vi "PDLM_DecodeLHFeatures.vi"(8 "error in (no error)":errorcluster, 10 "features":u32) -> (0 "error out":errorcluster, 2 "Buffer":string, 3 "return type":i32)   [LabVIEW 2019]
uses:
  <userlib>/TaikoLaser/PDLM_DllPath_global.vi
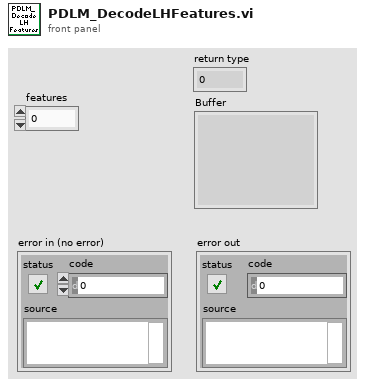
[diagram p1: front panel]
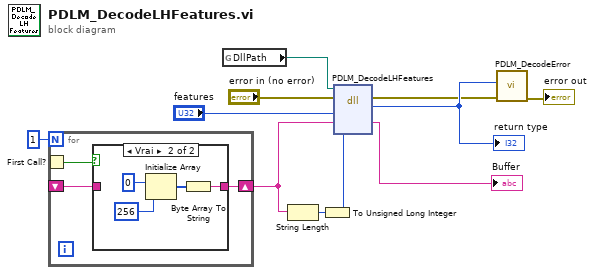
[diagram p0: block diagram]
diagram:
  n1 = for {
    N: 1 -> [_]
    shift-right: [w13] -> w1
    shift-left: _ -> [w12]
    n2 = First Call?() -> (First Call?: T/F=w14:bool)
    n3 = case shown="Vrai" w14 {
      tunnel: [w15 w16] -> w13
      tunnel: w12 -> [w15 _]
      frame False {
      }
      frame True {
        n4 = Initialize Array(u8 0, 256 ("dimension size")) -> (w17:u8[])
        n5 = Byte Array To String(unsigned byte array=w17) -> (string=w16:string)
      }
    }
  }
  n6 = global read "PDLM_DllPath_global.vi" "DllPath"() -> (w7:path)
  n7 = String Length(string=w1) -> (length=w6:i32)
  n8 = To Unsigned Long Integer(number=w6) -> (unsigned 32bit integer=w4:u32)
  n9 = dll-call lib="M:/_dev/progs/LabVIEW/_lib/PQ/Taiko/pdlm_lib.dll" fn="PDLM_DecodeLHFeatures"(path in=w7, error in="error in (no error)", "features"="features", "Buffer"=w1, "BuffLen"=w4) -> (error out=w9:errorcluster, "return type"=w10:i32, "Buffer"=→"Buffer":string)  [unwired: 3 in, 1 out]
  "return type" <- w10
  n10 = call <userlib>:"PDLM_DecodeError.vi"("error in (no error)"=w9, "code"=w10) -> ("error out"=→"error out":errorcluster)  [unwired: 7 in, 2 out]
